vi "High TC Interface.vi"() -> ()   [LabVIEW 2018]
uses:
  <vilib>/Utility/file.llb/Write Delimited Spreadsheet (DBL).vi
panel:
  out "R_sc (Ohms)":dbl
  out "Current (Amps)":dbl
  out "Voltage (Volts)":dbl
  out "Temperature (K)":dbl
  out "Temp v Resistance":cluster{"x":dbl, "y":dbl}[](graph)
  out "Elapsed Time (s)":dbl
  out "Temp Vs Time":cluster{"x":dbl, "y":dbl}[](graph)
  out "Resistance Vs Time":cluster{"x":dbl, "y":dbl}[](graph)
  in  "stop":bool
  # "Top"
  # "Bottom"
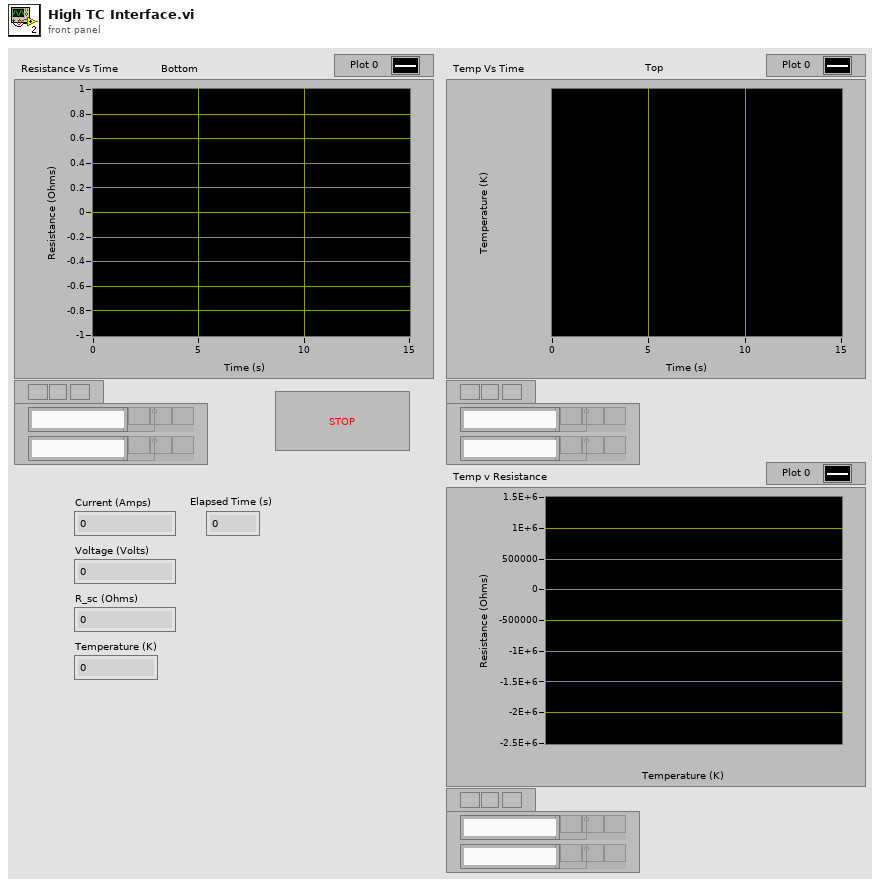
[diagram p1: front panel]
types:
  T1 = cluster{"Elapsed Time (s)":dbl, "Resistance(Therm)":dbl}
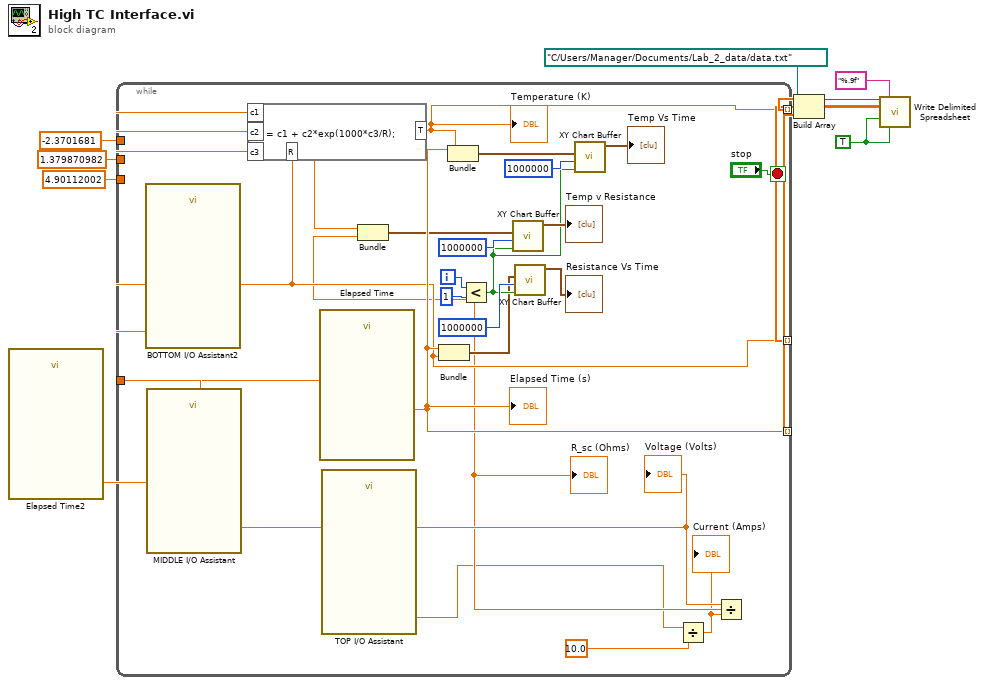
[diagram p0: block diagram]
diagram:
  w2 = TRUE ("transpose? (F)")
  n1 = call "Elapsed Time2"() -> ("Present (s)"=w11:dbl)  [unwired: 12 in, 7 out]
  n2 = while {
    tunnel: w11 -> [w32]
    tunnel: [w19] -> w9 mode=indexing
    tunnel: [w29] -> w8 mode=indexing
    tunnel: [w20] -> w7 mode=indexing
    tunnel: -2.3701681 -> [w18]
    tunnel: 1.379870982 -> [w17]
    tunnel: 4.90112002 -> [w16]
    i -> [w27]
    stop <- "stop" stop-if-true
    n3 = call "BOTTOM I/O Assistant2"() -> ("Resistance(Therm)"=w20:dbl)  [unwired: 25 in, 2 out]
    n4 = call "MIDDLE I/O Assistant"() -> ("Voltage"=w21:dbl)  [unwired: 25 in, 2 out]
    "Voltage (Volts)" <- w21
    n5 = formula code="T = c1 + c2*exp(1000*c3/R);"("c1"=w18, "c2"=w17, "c3"=w16, "R"=w20) -> ("T"=w19:dbl)
    "Temperature (K)" <- w19
    n6 = call "Elapsed Time"("Set Start Time (s)"=w32) -> ("Elapsed Time (s)"=w29:dbl)  [unwired: 11 in, 7 out]
    "Elapsed Time (s)" <- w29
    n7 = call "TOP I/O Assistant"() -> ("Current"=w12:dbl)  [unwired: 25 in, 2 out]
    n8 = Bundle("Elapsed Time (s)"=w29, "Resistance(Therm)"=w20) -> (w22:T1)  [unwired: 1 in]
    n9 = Bundle("Elapsed Time (s)"=w29, "T"=w19) -> (w30:cluster{"Elapsed Time (s)":dbl, "T":dbl})  [unwired: 1 in]
    n10 = Less?(x=w27, y=1) -> (x < y?=w24:bool)
    n11 = call "XY Chart Buffer.vi"("clear first (no:F)"=w24, "chart length (points)"=1000000, "new point"=w22) -> ("XY chart data"=→"Resistance Vs Time":cluster{"x":dbl, "y":dbl}[])  [unwired: 8 in]
    n12 = call "XY Chart Buffer.vi"("clear first (no:F)"=w24, "chart length (points)"=1000000, "new point"=w30) -> ("XY chart data"=→"Temp Vs Time":cluster{"x":dbl, "y":dbl}[])  [unwired: 8 in]
    n13 = Divide(x=w12, y=10.0) -> (x/y=w13:dbl)
    "Current (Amps)" <- w13
    n14 = Divide(x=w21, y=w13) -> (x/y=w15:dbl)
    "R_sc (Ohms)" <- w15
    n15 = Bundle("T"=w19, w15) -> (w23:cluster{"T":dbl, dbl})  [unwired: 1 in]
    n16 = call "XY Chart Buffer.vi"("clear first (no:F)"=w24, "chart length (points)"=1000000, "new point"=w23) -> ("XY chart data"=→"Temp v Resistance":cluster{"x":dbl, "y":dbl}[])  [unwired: 8 in]
  }
  n17 = Build Array(w9, w7, w8) -> (w1:dbl[][])
  n18 = call-poly <vilib>:"Write Delimited Spreadsheet.vi"("file path (dialog if empty)"=path "C:/Users/Manager/Documents/Lab_2_data/data.txt", "format (%.3f)"="%.9f", "2D data"=w1, "append to file? (new file:F)"=w2, "transpose? (no:F)"=w2) -> ()  [unwired: 9 in, 2 out]
